vi "getCustomer.vi"(8 "error in (no error)":errorcluster, 10 "name":string, 11 "CustomerFactory in":refnum<class "CustomerFactory.lvclass">) -> (0 "error out":errorcluster, 2 "AbstractCustomer.lvclass":refnum<class "AbstractCustomer.lvclass">, 3 "CustomerFactory out":refnum<class "CustomerFactory.lvclass">)   [LabVIEW 2018, in "CustomerFactory.lvclass"]
uses:
  CustomerFactory.lvclass
  AbstractCustomer Class/AbstractCustomer.lvclass
  NullCustomer Class/NullCustomer.lvclass
  C:/Users/fflores/Documents/LabVIEW-Open-Projects/LabIVEW OOP Design Patterns/Null Object Pattern/AbstractCustomer Class/AbstractCustomer.lvclass
  RealCustomer Class/RealCustomer.lvclass
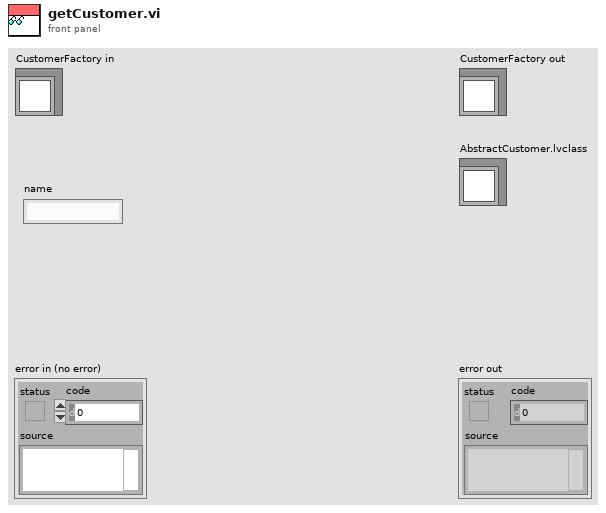
[diagram p1: front panel]
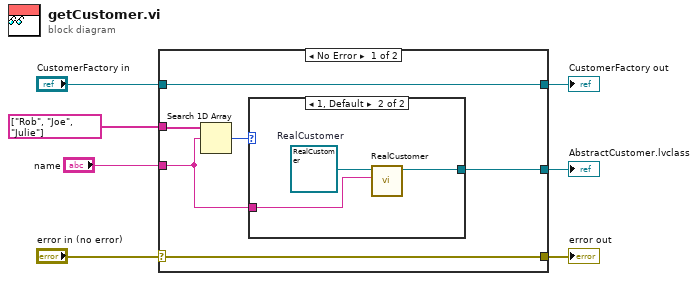
[diagram p0: block diagram]
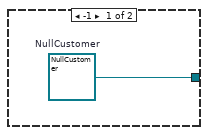
[diagram p2: hidden frame]
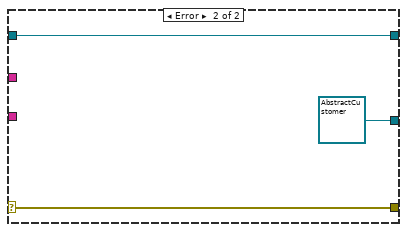
[diagram p3: hidden frame]
diagram:
  n1 = case shown="No Error" "error in (no error)" {
    selector: "error in (no error)" -> [w13 w19]
    tunnel: [w13 w19] -> w6
    tunnel: [w12 w20] -> w4
    tunnel: "CustomerFactory in" -> [w12 w20]
    tunnel: string[] ["Rob", "Joe", "Julie"] -> [w11 _]
    tunnel: "name" -> [w8 _]
    tunnel: [w9 refnum<class "AbstractCustomer.lvclass"> refnum ("AbstractCustomer.lvclass")] -> w1
    frame No Error {
      n2 = Search 1D Array(1D array=w11, element=w8) -> (index of element=w10:i32)  [unwired: 1 in]
      n3 = case shown="1, Default" w10 {
        tunnel: [w14 w16] -> w9
        tunnel: w8 -> [_ w15]
        frame -1 {
          w14 = refnum<class "NullCustomer.lvclass"> refnum  # NullCustomer
        }
        frame 1, Default {
          w17 = refnum<class "RealCustomer.lvclass"> refnum  # RealCustomer
          n4 = call "RealCustomer.vi"("name"=w15, "RealCustomer in"=w17) -> ("RealCustomer out"=w16:refnum<class "RealCustomer.lvclass">)  [unwired: 8 in, 1 out]
        }
      }
    }
    frame Error {
    }
  }
  "error out" <- w6
  "CustomerFactory out" <- w4
  "AbstractCustomer.lvclass" <- w1
